vi "Read Analog Input.vi"(8 "error in (no error)":errorcluster, 10 "Channel":i32, 11 "VISA resource name in":refnum<visa-resource-name>) -> (0 "error out":errorcluster, 1 "Value":u16, 3 "VISA resource name":refnum<visa-resource-name>)   [LabVIEW 2023, in "CTI-Visa.lvlib"]
uses:
  CTI-Visa.lvlib
  7fea3a05-604e-48c4-beb9-60477fbd2fb8.vi
  40ef9531-6e68-4b2d-bda6-0c1a52ee5349.vi
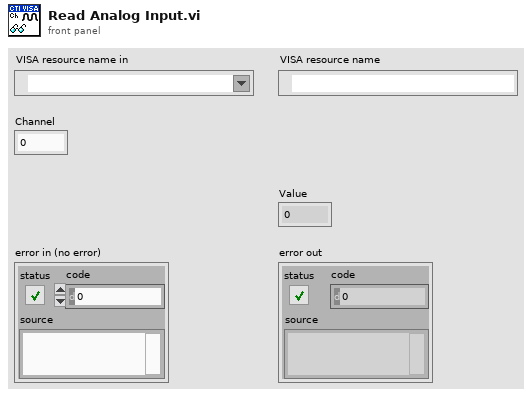
[diagram p1: front panel]
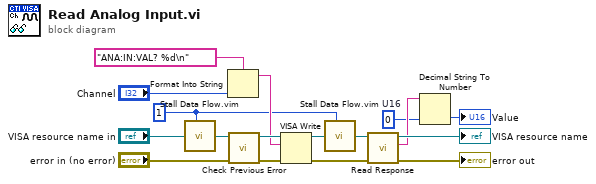
[diagram p0: block diagram]
diagram:
  w3 = u16 0  # U16
  w9 = u32 1 ("milliseconds to wait")
  n1 = call "Stall Data Flow.vim"("value in"="VISA resource name in", "milliseconds to wait"=w9) -> ("value out"=w11:refnum<visa-resource-name>)  [unwired: 1 out]
  n2 = Format Into String(format string="ANA:IN:VAL? %d\n", "Channel") -> (resulting string=w14:string)  [unwired: 2 in, 1 out]
  n3 = call "Check Previous Error.vi"("error in (no error)"="error in (no error)", "VISA resource name in"=w11) -> ("error out"=w15:errorcluster, "VISA resource name"=w16:refnum<visa-resource-name>)  [unwired: 8 in]
  n4 = VISA Write(VISA resource name=w16, write buffer=w14, error in (no error)=w15) -> (VISA resource name out=w13:refnum<visa-resource-name>, error out=w12:errorcluster)  [unwired: 1 out]
  n5 = call "Stall Data Flow.vim"("value in"=w13, "milliseconds to wait"=w9) -> ("value out"=w10:refnum<visa-resource-name>)  [unwired: 1 out]
  n6 = call "Read Response.vi"("error in (no error)"=w12, "VISA resource name in"=w10) -> ("error out"=→"error out":errorcluster, "Response"=w4:string, "VISA resource name"=→"VISA resource name":refnum<visa-resource-name>)  [unwired: 7 in]
  n7 = Decimal String To Number(string=w4, default (0L)=w3) -> (number=→"Value":u16)  [unwired: 1 in, 1 out]
